vi "Open APU Setup File.vi"(8 "error in":errorcluster, 10 "APUName":string, 11 "APUSetupFolder":path) -> (0 "error out":errorcluster, 1 "APUSetupFile":path, 3 "APU Setup File":T1)   [LabVIEW 2018, in "File IO.lvlib"]
uses:
  File IO.lvlib
  Top Level/Shared Controls/APU Setup File.ctl
  <vilib>/Utility/NIReport.llb/Report Type.ctl
  <vilib>/addons/_office/excel.llb/Excel Get Data ([str]).vi
  <vilib>/Utility/NIReport.llb/NI_report.lvclass
  <vilib>/Utility/NIReport.llb/Excel/NI_Excel.lvclass
  <vilib>/addons/_office/NI_ReportGenerationToolkit.lvlib
  <vilib>/Utility/NIReport.llb/NI_ReportGenerationCore.lvlib
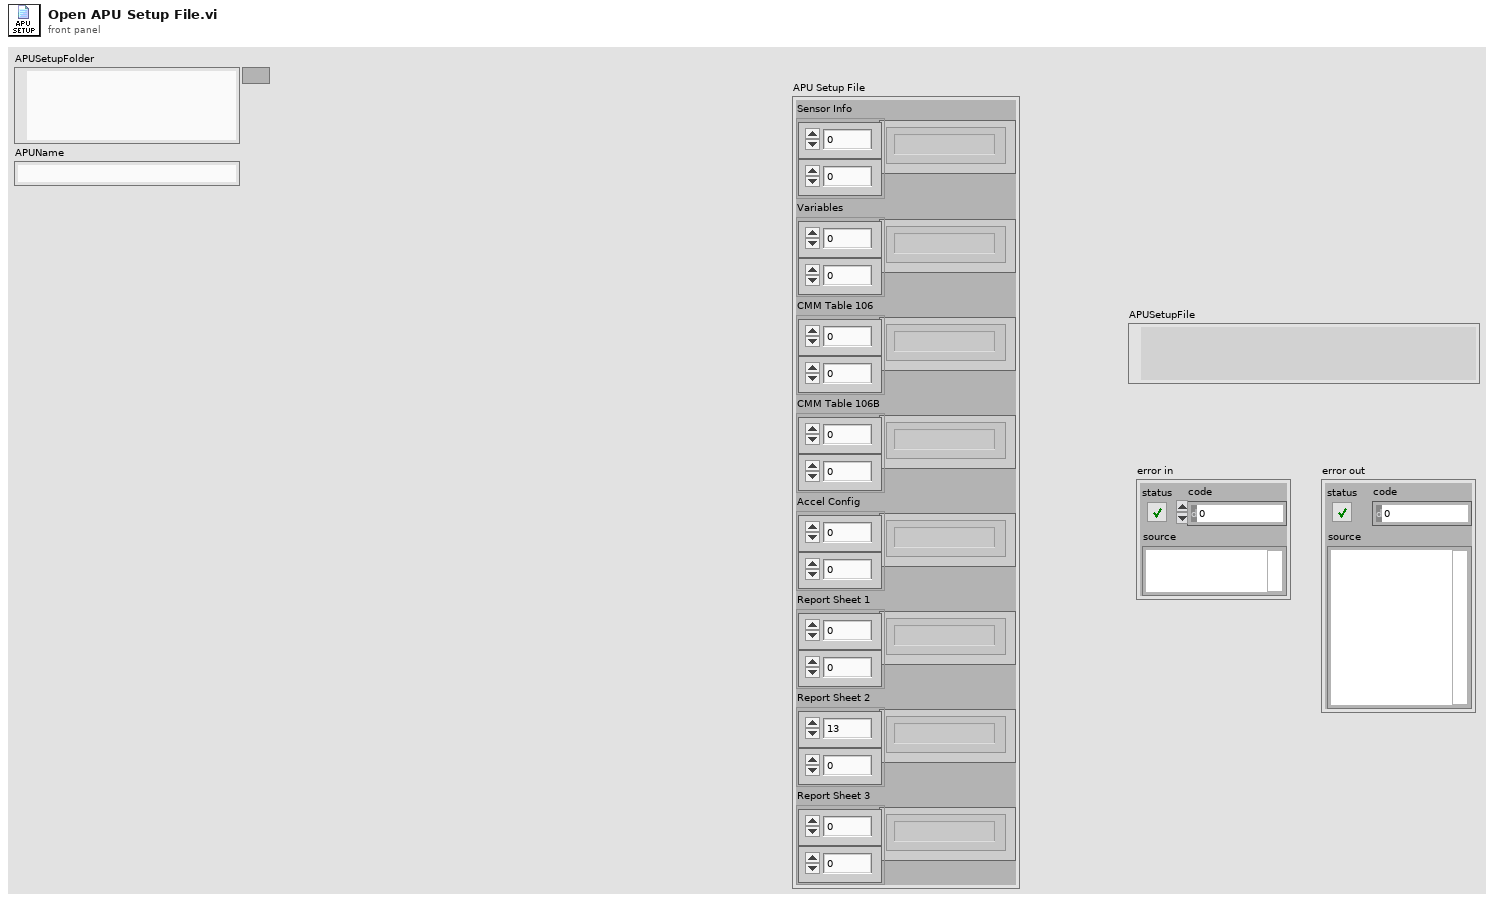
[diagram p1: front panel]
types:
  T1 = typedef "APU Setup File.ctl" = cluster{"Sensor Info":string[][], "Variables":string[][], "CMM Table 106":string[][], "CMM Table 106B ":string[][], "Accel Config":string[][], "Report Sheet 1":string[][], "Report Sheet 2":string[][], "Report Sheet 3":string[][]}
  T2 = typedef "NI_ReportGenerationCore.lvlib/Report Type.ctl" = enum16{"HTML", "Word", "Excel"}
  T3 = enum16{"maximized", "minimized", "normal", "no change"}
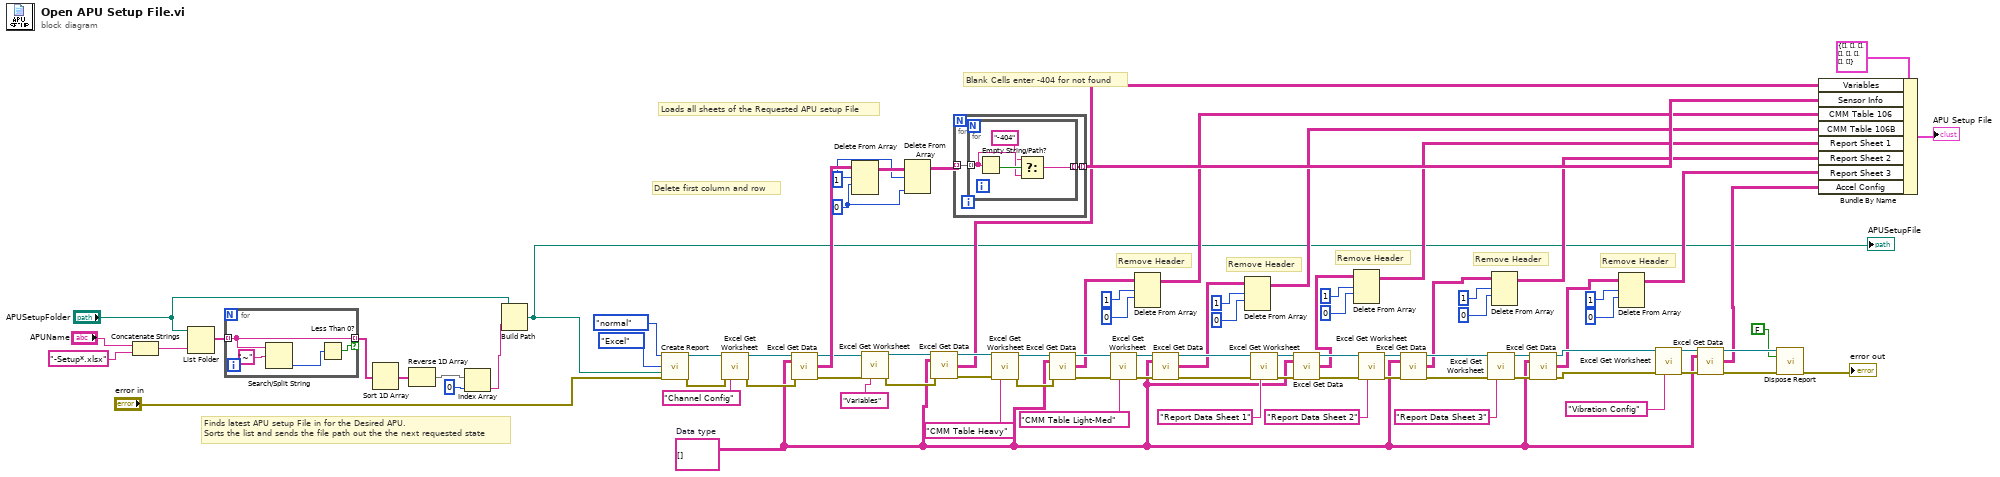
[diagram p0: block diagram]
diagram:
  w6 = string[][] []  # Data type
  w78 = 1 ("length")
  w77 = 0 ("index (row)")
  # "Remove Header"
  # "Remove Header"
  # "Remove Header"
  # "Remove Header"
  # "Remove Header"
  # "Delete first column and row"
  # "Blank Cells enter -404 for not found"
  # "Loads all sheets of the Requested APU setup File"
  # "Finds latest APU setup File in for the Desired APU. \nSorts the list and sends the file path out the the next requested state"
  n1 = Concatenate Strings("APUName", "-Setup*.xlsx" ("pattern")) -> (w81:string)
  n2 = List Folder(path="APUSetupFolder", pattern=w81) -> (filenames=w86:string[])  [unwired: 2 in, 3 out]
  n3 = for {
    tunnel: w86 -> [w93] mode=indexing
    tunnel: [w93] -> w87 mode=indexing if=w91
    n4 = Search/Split String(string=w93, search string/char (-)="~") -> (offset of match=w90:i32)  [unwired: 1 in, 2 out]
    n5 = Less Than 0?(x=w90) -> (x < 0?=w91:bool)
  }
  n6 = Sort 1D Array(array=w87) -> (sorted array=w85:string[])
  n7 = Reverse 1D Array(array=w85) -> (reversed array=w84:string[])
  n8 = Index Array(array=w84, index=0) -> (element=w1:string)
  n9 = Build Path(base path="APUSetupFolder", name or relative path=w1) -> (appended path=w2:path)
  "APUSetupFile" <- w2
  n10 = call <vilib>:"Create Report.vi"("window state (normal)"=T3."normal", "report type"=Report_Type."Excel", "template (empty)"=w2, "error in (no error)"="error in") -> ("report out"=w69:refnum<class "NI_report.lvclass">, "error out"=w68:errorcluster)  [unwired: 10 in]
  n11 = call <vilib>:"Excel Get Worksheet.vi"("report in"=w69, "error in (no error)"=w68, "name (\"\")"="Channel Config" ("name (\"\")")) -> ("report out"=w71:refnum<class "NI_report.lvclass">, "error out"=w72:errorcluster)  [unwired: 11 in]
  n12 = call-poly <vilib>:"Excel Get Data.vi"("report in"=w71, "data type"=w6, "error in (no error)"=w72) -> ("report out"=w10:refnum<class "NI_report.lvclass">, "data"=w80:string[][], "error out"=w9:errorcluster)  [unwired: 10 in]
  n13 = Delete From Array(array=w80, length=w78, index (row)=w77) -> (array with subset deleted=w79:string[][])  [unwired: 1 in, 1 out]
  n14 = call <vilib>:"Excel Get Worksheet.vi"("report in"=w10, "error in (no error)"=w9, "name (\"\")"="Variables" ("name (\"\")")) -> ("report out"=w12:refnum<class "NI_report.lvclass">, "error out"=w13:errorcluster)  [unwired: 11 in]
  n15 = Delete From Array(array=w79, length=w78, index (col)=w77) -> (array with subset deleted=w76:string[][])  [unwired: 1 in, 1 out]
  n16 = call-poly <vilib>:"Excel Get Data.vi"("report in"=w12, "data type"=w6, "error in (no error)"=w13) -> ("report out"=w7:refnum<class "NI_report.lvclass">, "data"=w5:string[][], "error out"=w8:errorcluster)  [unwired: 10 in]
  n17 = for {
    tunnel: w76 -> [w95] mode=indexing
    tunnel: [w94] -> w74 mode=indexing
    n18 = for {
      tunnel: w95 -> [w98] mode=indexing
      tunnel: [w96] -> w94 mode=indexing
      n19 = Empty String/Path?(string/path=w98) -> (empty?=w99:bool)
      n20 = Select(t="-404", s=w99, f=w98) -> (s? t:f=w96:string)
    }
  }
  n21 = call <vilib>:"Excel Get Worksheet.vi"("report in"=w7, "error in (no error)"=w8, "name (\"\")"="CMM Table Heavy" ("name (\"\")")) -> ("report out"=w66:refnum<class "NI_report.lvclass">, "error out"=w67:errorcluster)  [unwired: 11 in]
  n22 = call-poly <vilib>:"Excel Get Data.vi"("report in"=w66, "data type"=w6, "error in (no error)"=w67) -> ("report out"=w65:refnum<class "NI_report.lvclass">, "data"=w21:string[][], "error out"=w64:errorcluster)  [unwired: 10 in]
  n23 = call <vilib>:"Excel Get Worksheet.vi"("report in"=w65, "error in (no error)"=w64, "name (\"\")"="CMM Table Light-Med" ("name (\"\")")) -> ("report out"=w61:refnum<class "NI_report.lvclass">, "error out"=w62:errorcluster)  [unwired: 11 in]
  n24 = Delete From Array(array=w21, length=1 ("disabled index (col)"), index (row)=0) -> (array with subset deleted=w20:string[][])  [unwired: 1 in, 1 out]
  n25 = call-poly <vilib>:"Excel Get Data.vi"("report in"=w61, "data type"=w6, "error in (no error)"=w62) -> ("report out"=w55:refnum<class "NI_report.lvclass">, "data"=w17:string[][], "error out"=w54:errorcluster)  [unwired: 10 in]
  n26 = Delete From Array(array=w17, length=1 ("disabled index (col)"), index (row)=0) -> (array with subset deleted=w16:string[][])  [unwired: 1 in, 1 out]
  n27 = call <vilib>:"Excel Get Worksheet.vi"("report in"=w55, "error in (no error)"=w54, "name (\"\")"="Report Data Sheet 1" ("name (\"\")")) -> ("report out"=w57:refnum<class "NI_report.lvclass">, "error out"=w56:errorcluster)  [unwired: 11 in]
  n28 = call-poly <vilib>:"Excel Get Data.vi"("report in"=w57, "data type"=w6, "error in (no error)"=w56) -> ("report out"=w36:refnum<class "NI_report.lvclass">, "data"=w35:string[][], "error out"=w40:errorcluster)  [unwired: 10 in]
  n29 = Delete From Array(array=w35, length=1 ("disabled index (col)"), index (row)=0) -> (array with subset deleted=w51:string[][])  [unwired: 1 in, 1 out]
  n30 = call <vilib>:"Excel Get Worksheet.vi"("report in"=w36, "error in (no error)"=w40, "name (\"\")"="Report Data Sheet 2" ("name (\"\")")) -> ("report out"=w34:refnum<class "NI_report.lvclass">, "error out"=w39:errorcluster)  [unwired: 11 in]
  n31 = call-poly <vilib>:"Excel Get Data.vi"("report in"=w34, "data type"=w6, "error in (no error)"=w39) -> ("report out"=w33:refnum<class "NI_report.lvclass">, "data"=w30:string[][], "error out"=w38:errorcluster)  [unwired: 10 in]
  n32 = call <vilib>:"Excel Get Worksheet.vi"("report in"=w33, "error in (no error)"=w38, "name (\"\")"="Report Data Sheet 3" ("name (\"\")")) -> ("report out"=w32:refnum<class "NI_report.lvclass">, "error out"=w42:errorcluster)  [unwired: 11 in]
  n33 = Delete From Array(array=w30, length=1 ("disabled index (col)"), index (row)=0) -> (array with subset deleted=w29:string[][])  [unwired: 1 in, 1 out]
  n34 = call-poly <vilib>:"Excel Get Data.vi"("report in"=w32, "data type"=w6, "error in (no error)"=w42) -> ("report out"=w41:refnum<class "NI_report.lvclass">, "data"=w25:string[][], "error out"=w37:errorcluster)  [unwired: 10 in]
  n35 = Delete From Array(array=w25, length=1 ("disabled index (col)"), index (row)=0) -> (array with subset deleted=w24:string[][])  [unwired: 1 in, 1 out]
  n36 = call <vilib>:"Excel Get Worksheet.vi"("report in"=w41, "error in (no error)"=w37, "name (\"\")"="Vibration Config" ("name (\"\")")) -> ("report out"=w50:refnum<class "NI_report.lvclass">, "error out"=w49:errorcluster)  [unwired: 11 in]
  n37 = call-poly <vilib>:"Excel Get Data.vi"("report in"=w50, "data type"=w6, "error in (no error)"=w49) -> ("report out"=w46:refnum<class "NI_report.lvclass">, "data"=w45:string[][], "error out"=w48:errorcluster)  [unwired: 10 in]
  n38 = call-dynamic "Dispose Report.vi"("report in"=w46, "wait until printing completed? (T)"=FALSE, "error in (no error)"=w48) -> ("error out"=→"error out":errorcluster)  [unwired: 12 in]
  n39 = Bundle By Name(cluster=T1 {"Sensor Info"=[], "Variables"=[], "CMM Table 106"=[], "CMM Table 106B "=[], "Accel Config"=[], "Report Sheet 1"=[], "Report Sheet 2"=[], "Report Sheet 3"=[]} ("APU Setup File"), "Variables"=w5, "Sensor Info"=w74, "CMM Table 106"=w20, "CMM Table 106B"=w16, "Report Sheet 1"=w51, "Report Sheet 2"=w29, "Report Sheet 3"=w24, "Accel Config"=w45) -> (→"APU Setup File":T1)
